vi "Clear Bundle Definitions Tree.vi"(8 "error in":errorcluster, 11 "TreeControl in":refnum<vi>) -> (0 "error out":errorcluster, 3 "TreeControl out":refnum<vi>)   [LabVIEW 2020]
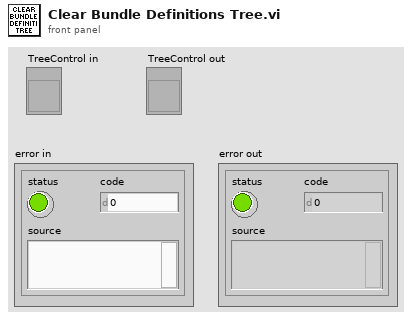
[diagram p1: front panel]
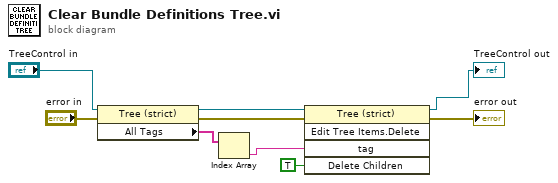
[diagram p0: block diagram]
diagram:
  n1 = property class="Tree (strict)"(reference="TreeControl in", error in="error in") -> (reference out=w9:refnum<vi>, error out=w6:errorcluster, "All Tags"=w3:string[])
  n2 = Index Array(array=w3) -> (element=w2:string)  [unwired: 1 in]
  n3 = invoke class="Tree (strict)" method="Edit Tree Items.Delete"(reference=w9, error in=w6, "tag"=w2, "Delete Children"=TRUE ("Delete Children?")) -> (reference out=→"TreeControl out":refnum<vi>, error out=→"error out":errorcluster)  [unwired: 1 in, 3 out]
